vi "Ass IO Status.vi"(8 "error in (no error)":errorcluster) -> (0 "error out":errorcluster)   [LabVIEW 2017]
uses:
  <vilib>/NI/Modbus Library/API/Wrapper/Create TCP Master.vi
  <vilib>/NI/Modbus Library/API/master/Modbus Master.lvclass
  <vilib>/NI/Modbus Library/API/Wrapper/API Main.lvlib
panel:
  in  "Tab Control":enum32{"INPUTS", "OUTPUTS"}(tab)
  out "SPARE 10":bool
  out "SPARE 9":bool
  out "SPARE 8":bool
  out "SPARE 7":bool
  out "SPARE 6":bool
  out "SPARE 5":bool
  out "SPARE 3":bool
  out "SPARE 4":bool
  out "LH TILT SLIDE POSITION - X40":bool
  out "RH TILT SLIDE POSITION - X41":bool
  out "SPARE 1":bool
  out "SPARE 2":bool
  out "REJECTION BOX - X37":bool
  out "LH FIXTURE POSSITION - X33":bool
  out "RH FIXTURE POSSITION - X34":bool
  out "RH MECH SLIDE POSSITION - X35":bool
  out "LH MECH SLIDE POSSITION - X36":bool
  out "EMERGENCY E-STOP - X0":bool
  out "Cycle Start PB 1- X1":bool
  out "Reset PB - X2":bool
  out "Cycle Start PB 2- X3":bool
  out "TILT SENSOR UP - X4":bool
  out "TILT SENSOR UP - X5":bool
  out "VACCUME DOWN - X6":bool
  out "VACCUME UP - X7":bool
  out "AIR PRESSURE 1 - X20":bool
  out "VACCUME MID - X21":bool
  out "TILT SR SLID HOME - X22":bool
  out "TILT SR SLID FRD - X23":bool
  out "CLAMP HOME - X24":bool
  out "AIR PRESSURE 2 - X25":bool
  out "JOYSTICK X1 DOWN CLOSE - X26":bool
  out "JOYSTICK Y1 DOWN OPEN - X27":bool
  out "JOYSTICK X2 DOWN CLOSE - X30":bool
  out "JOYSTICK Y2 DOWN OPEN - X31":bool
  out "PUNCH - X32":bool
  in  "DECLAMP - Y0":bool
  in  "CLAMP - Y1":bool
  in  "TILT SR CYL SLID FRD - Y2":bool
  in  "TILT SR CYL SLID REV - Y3":bool
  in  "SPARE":bool
  in  "SPARE":bool
  in  "SPARE":bool
  in  "SPARE":bool
  in  "AIR ON UP AND DOWN - Y20":bool
  in  "ROTATING CYL - Y21":bool
  in  "PUNCH - Y23":bool
  in  "X-Y JOYSTICK CYL UP - Y24":bool
  in  "X-Y JOYSTICK CYL DW - Y25":bool
  in  "VACCUME UP/DOWM - Y26":bool
  in  "VACCUME - Y27":bool
  in  "SPARE":bool
  in  "RED TOWER LAMP - Y31":bool
  in  "YELLOW TOWER LAMP - Y32":bool
  in  "GREEN TOWER LAMP - Y33":bool
  in  "POLARITY - Y34":bool
  in  "MOTOR 2 - Y36":bool
  in  "SPARE":bool
  in  "SPARE":bool
  in  "SPARE":bool
  in  "SPARE":bool
  in  "SPARE":bool
  in  "SPARE":bool
  in  "SPARE":bool
  in  "SPARE":bool
  in  "SPARE":bool
  in  "ROTATING CYL HOME - Y22":bool
  in  "MOTOR 1 - Y35":bool
  in  "SPARE":bool
  in  "stop":bool
  # "LEAKTEST STATION IO STATUS"
  # "ASSEMBLY STATION IO STATUS"
  # "RBC ORVM STATION IO STATUS"
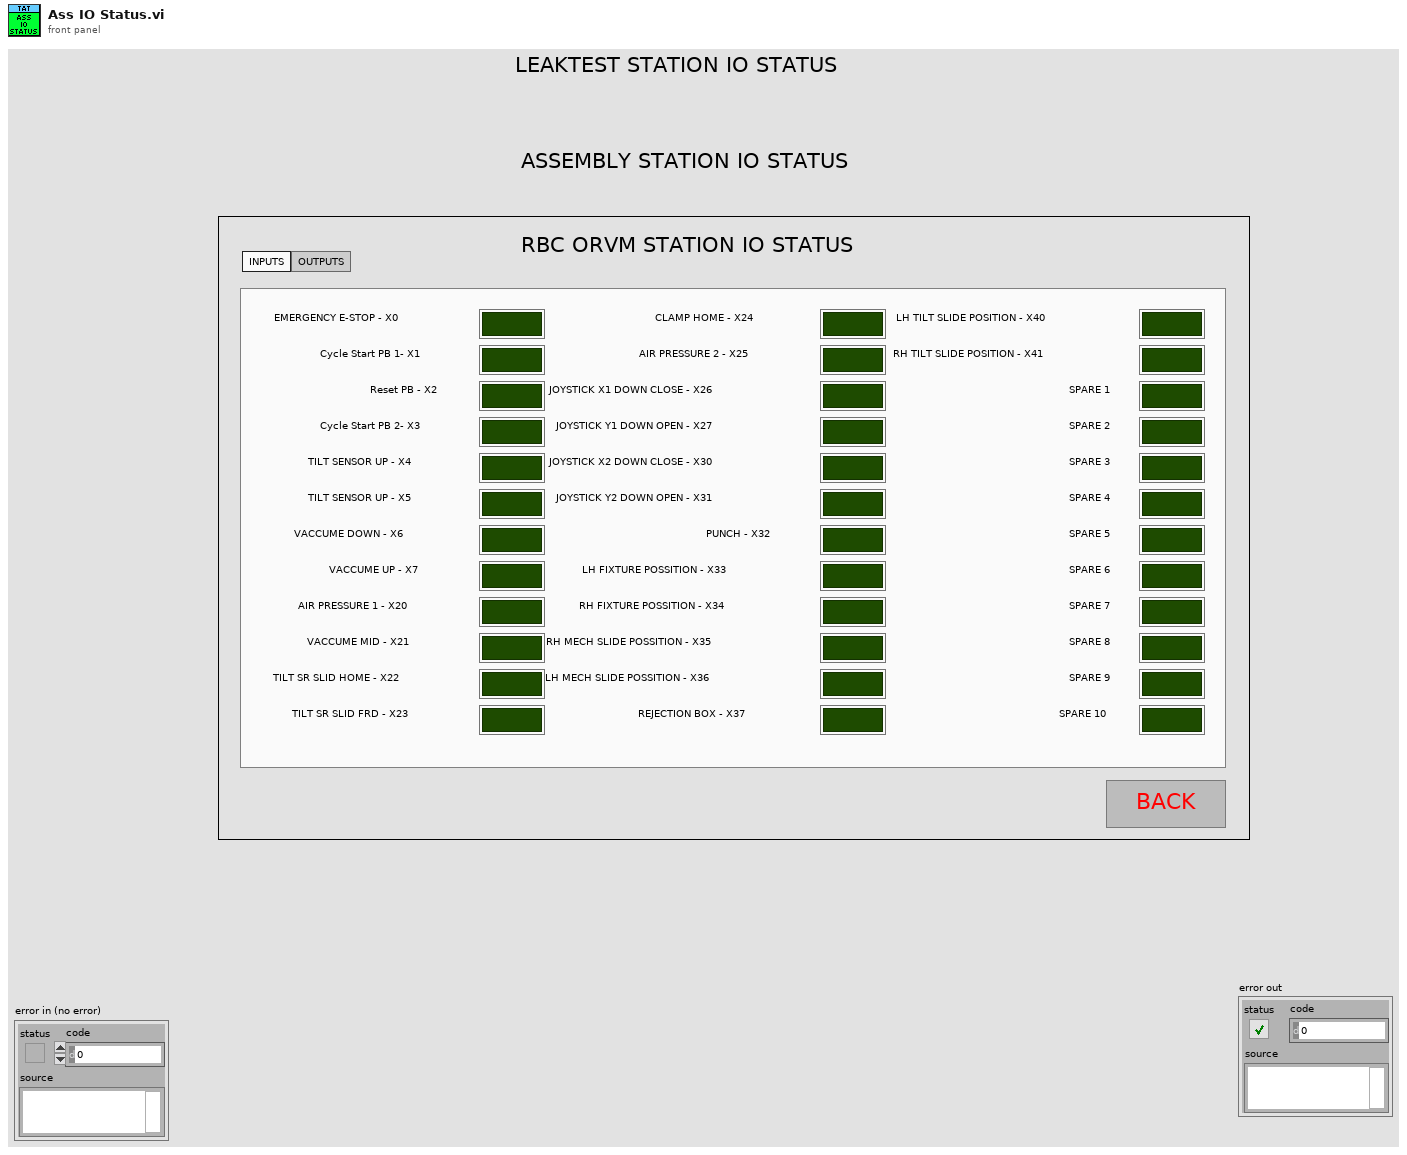
[diagram p1: front panel]
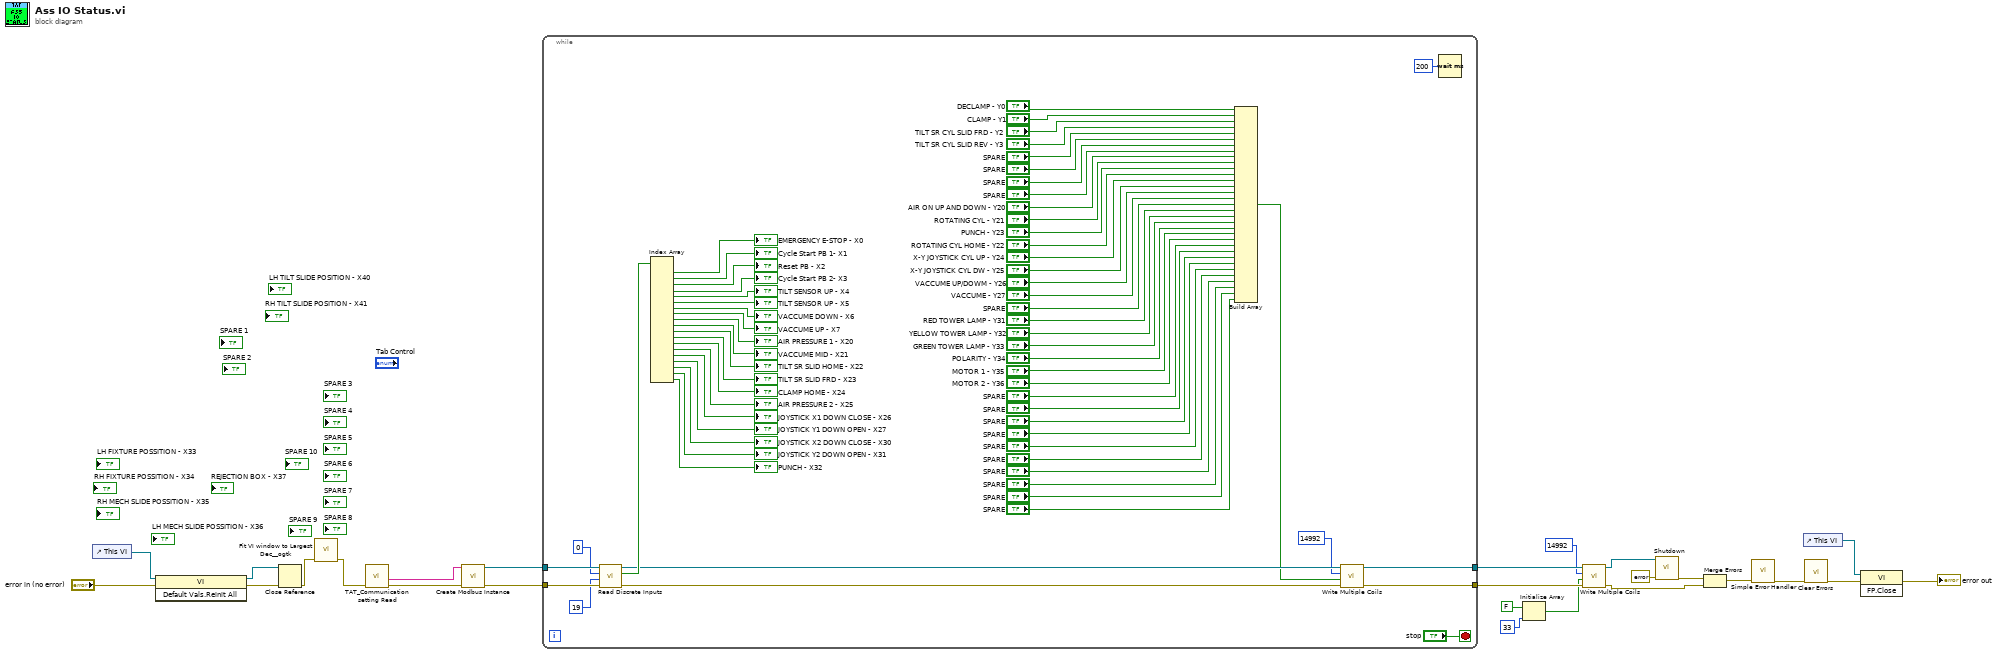
[diagram p0: block diagram]
diagram:
  n1 = control-ref of="This VI"() -> (w6:refnum<vi>)
  n2 = invoke class="VI" method="Default Vals.Reinit All"(reference=w6, error in="error in (no error)") -> (reference out=w4:refnum<vi>, error out=w3:errorcluster)  [unwired: 1 in, 1 out]
  n3 = Close Reference(reference=w4, error in (no error)=w3) -> (error out=w2:errorcluster)
  n4 = call <userlib>:"Fit VI window to Largest Dec__ogtk.vi"("error in (no error)"=w2) -> ("error out"=w1:errorcluster)  [unwired: 5 in, 1 out]
  n5 = call "TAT_Communication setting Read.vi"("error in (no error)"=w1) -> ("error out"=w25:errorcluster, "PLC IP"=w24:string)  [unwired: 3 in, 6 out]
  n6 = call-poly <vilib>:"Create Modbus Instance.vi"("error in"=w25, "address"=w24) -> ("error out"=w23:errorcluster, "TCP master instance"=w22:refnum<class "Modbus Master.lvclass">)  [unwired: 8 in]
  n7 = while {
    tunnel: w23 -> [w89]
    tunnel: w22 -> [w88]
    tunnel: [w27] -> w12
    tunnel: [w26] -> w14
    stop <- "stop" stop-if-true
    n8 = call-dynamic "Read Discrete Inputs.vi"("error in"=w89, "number of inputs"=u16 19, "starting address"=u16 0, "Modbus master in"=w88) -> ("error out"=w63:errorcluster, "discrete inputs"=w85:bool[], "Modbus master out"=w64:refnum<class "Modbus Master.lvclass">)  [unwired: 5 in]
    n9 = Index Array(array=w85) -> (element #1=→"EMERGENCY E-STOP - X0":bool, element #2=→"Cycle Start PB 1- X1":bool, element #3=→"Reset PB - X2":bool, element #4=→"Cycle Start PB 2- X3":bool, element #5=→"TILT SENSOR UP - X4":bool, element #6=→"TILT SENSOR UP - X5":bool, element #7=→"VACCUME DOWN - X6":bool, element #8=→"VACCUME UP - X7":bool, element #9=→"AIR PRESSURE 1 - X20":bool, element #10=→"VACCUME MID - X21":bool, element #11=→"TILT SR SLID HOME - X22":bool, element #12=→"TILT SR SLID FRD - X23":bool, element #13=→"CLAMP HOME - X24":bool, element #14=→"AIR PRESSURE 2 - X25":bool, element #15=→"JOYSTICK X1 DOWN CLOSE - X26":bool, element #16=→"JOYSTICK Y1 DOWN OPEN - X27":bool, element #17=→"JOYSTICK X2 DOWN CLOSE - X30":bool, element #18=→"JOYSTICK Y2 DOWN OPEN - X31":bool, element #19=→"PUNCH - X32":bool)  [unwired: 19 in]
    n10 = Build Array("DECLAMP - Y0", "CLAMP - Y1", "TILT SR CYL SLID FRD - Y2", "TILT SR CYL SLID REV - Y3", "SPARE", "SPARE", "SPARE", "SPARE", "AIR ON UP AND DOWN - Y20", "ROTATING CYL - Y21", "PUNCH - Y23", "ROTATING CYL HOME - Y22", "X-Y JOYSTICK CYL UP - Y24", "X-Y JOYSTICK CYL DW - Y25", "VACCUME UP/DOWM - Y26", "VACCUME - Y27", "SPARE", "RED TOWER LAMP - Y31", "YELLOW TOWER LAMP - Y32", "GREEN TOWER LAMP - Y33", "POLARITY - Y34", "MOTOR 1 - Y35", "MOTOR 2 - Y36", "SPARE", "SPARE", "SPARE", "SPARE", "SPARE", "SPARE", "SPARE", "SPARE", "SPARE", "SPARE") -> (w28:bool[])
    n11 = call-dynamic "Write Multiple Coils.vi"("error in"=w63, "coils to write"=w28, "starting address"=u16 14992, "Modbus master in"=w64) -> ("error out"=w27:errorcluster, "Modbus master out"=w26:refnum<class "Modbus Master.lvclass">)  [unwired: 6 in]
    n12 = Wait (ms)(milliseconds to wait=u32 200) -> ()  [unwired: 1 out]
  }
  n13 = Initialize Array(FALSE, 33 ("dimension size")) -> (w7:bool[])
  n14 = call-dynamic "Write Multiple Coils.vi"("error in"=w12, "coils to write"=w7, "starting address"=u16 14992, "Modbus master in"=w14) -> ("error out"=w11:errorcluster, "Modbus master out"=w13:refnum<class "Modbus Master.lvclass">)  [unwired: 6 in]
  n15 = call-dynamic "Shutdown.vi"("error in"=errorcluster {"status"=FALSE, "code"=0, "source"=""}, "Modbus master in"=w13) -> ("error out"=w20:errorcluster)  [unwired: 9 in]
  n16 = Merge Errors(w20, w11) -> (w19:errorcluster)
  n17 = call <vilib>:"Simple Error Handler.vi"("error in (no error)"=w19) -> ("error out"=w18:errorcluster)  [unwired: 4 in, 4 out]
  n18 = control-ref of="This VI"() -> (w16:refnum<vi>)
  n19 = call <vilib>:"Clear Errors.vi"("error in (no error)"=w18) -> ("error out"=w17:errorcluster)  [unwired: 5 in, 1 out]
  n20 = invoke class="VI" method="FP.Close"(reference=w16, error in=w17) -> (error out=→"error out":errorcluster)  [unwired: 1 in, 2 out]
